vi "decode-readdata.vi"(0 "字符串输入":string) -> (1 "有无后续帧":bool, 2 "数据处理状态":bool, 3 "数据字符串":string, 4 "类型字符串":string)   [LabVIEW 2010]
panel:
  out "字符串输入 2":string
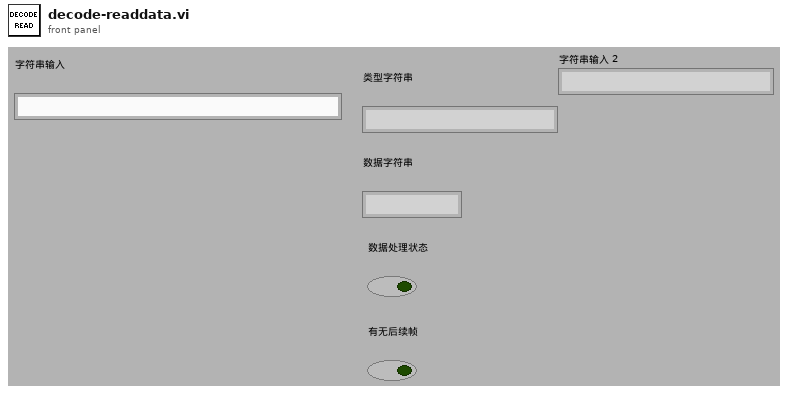
[diagram p1: front panel]
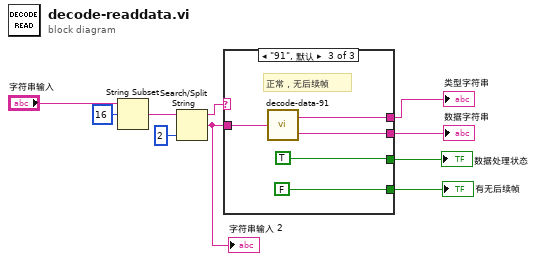
[diagram p0: block diagram]
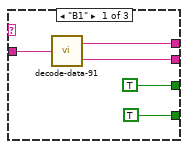
[diagram p2: hidden frame]
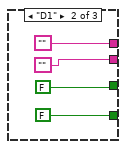
[diagram p3: hidden frame]
diagram:
  n1 = String Subset(string="字符串输入", offset (0)=16 ("偏移量(0)")) -> (substring=w4:string)  [unwired: 1 in]
  n2 = Search/Split String(string=w4, offset (0)=2 ("偏移量(0)")) -> (substring before match=w6:string, match + rest of string=w1:string)  [unwired: 1 in, 1 out]
  "字符串输入 2" <- w1
  n3 = case shown="\"91\", 默认" w6 {
    tunnel: w1 -> [w15 _ w24]
    tunnel: [w14 "" w23] -> w7
    tunnel: [w13 "" w22] -> w8
    tunnel: [TRUE FALSE TRUE] -> w9
    tunnel: [TRUE FALSE FALSE] -> w10
    frame "B1" {
      n4 = call "decode-data-91.vi"("输入字符串"=w15) -> ("数据字符串"=w13:string, "类型字符串"=w14:string)
    }
    frame "D1" {
    }
    frame "91", Default {
      # "正常，无后续帧"
      n5 = call "decode-data-91.vi"("输入字符串"=w24) -> ("数据字符串"=w22:string, "类型字符串"=w23:string)
    }
  }
  "有无后续帧" <- w10
  "数据处理状态" <- w9
  "数据字符串" <- w8
  "类型字符串" <- w7
